vi "getThrust.vi"(8 "error in (no error)":errorcluster, 10 "Throttle % [0-100]":dbl, 11 "OHAUS AV8101 in":refnum<class "OHAUS AV8101.lvclass">) -> (0 "error out":errorcluster, 2 "Thrust [g]":dbl, 3 "OHAUS AV8101 out":refnum<class "OHAUS AV8101.lvclass">)   [LabVIEW 2015, in "OHAUS AV8101.lvclass"]
uses:
  OHAUS AV8101.lvclass
  OHAUS AV8101.lvclass/OHAUS AV8101.ctl
  OHAUS AV8101 Drivers/Ohaus AV Series.lvlib
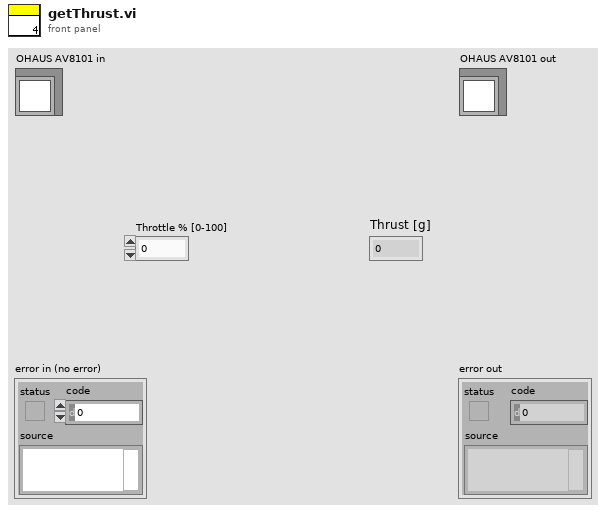
[diagram p1: front panel]
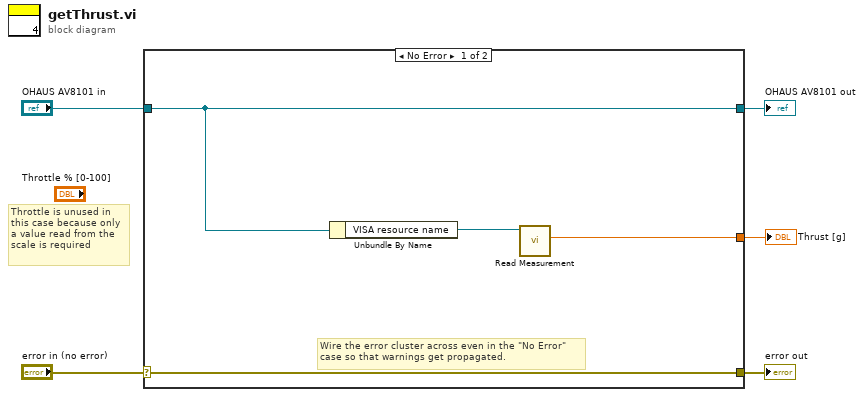
[diagram p0: block diagram]
diagram:
  # "Throttle is unused in\nthis case because only\na value read from the \nscale is required"
  n1 = case shown="No Error" "error in (no error)" {
    selector: "error in (no error)" -> [w9 w11]
    tunnel: [w9 w11] -> w4
    tunnel: [w8 w10] -> w2
    tunnel: "OHAUS AV8101 in" -> [w8 w10]
    tunnel: [w6 _] -> w1
    frame No Error {
      # "Wire the error cluster across even in the \"No Error\"\ncase so that warnings get propagated."
      n2 = Unbundle By Name(w8) -> ("VISA resource name"=w7:refnum<visa-resource-name>)
      n3 = call "Read Measurement.vi"("VISA resource name"=w7) -> ("Weight Value"=w6:dbl)  [unwired: 5 in, 5 out]
    }
    frame Error {
    }
  }
  "error out" <- w4
  "OHAUS AV8101 out" <- w2
  "Thrust [g]" <- w1
